vi "bats.parser.test.Multiple.SequencedUnitHeader.vi"() -> (3 "Passed":bool)   [LabVIEW 2022 SP3]
uses:
  pitch/AddOrder/AddOrderLong.Parameters.ctl
  pitch/ModifyOrder/ModifyOrderLong.Parameters.ctl
  <vilib>/Utility/error.llb/Trim Whitespace One-Sided.vi
  pitch/SequencedUnitHeader/SequencedUnitHeader.lvclass
  pitch/MessageBase/MessageBase.lvclass
  pitch/AddOrder/AddOrderLong.lvclass
  pitch/ModifyOrder/ModifyOrderLong.lvclass
panel:
  in  "ModifyOrderLong.Parameters 2":T1={"Time Offset"=0, "Order Id"="OD03", "Quantity"=0, "Price"=0.0, "Modify Flags"=0}
  in  "AddOrderLong.Parameters 2":T2={"Time Offset"=0, "Order Id"="OD02", "Quantity"=0, "Symbol"="", "Side Indicator"="", "Price"=0.0}
  in  "ModifyOrderLong.Parameters":T1={"Time Offset"=0, "Order Id"="OD02", "Quantity"=0, "Price"=0.0, "Modify Flags"=0}
  in  "AddOrderLong.Parameters":T2={"Time Offset"=0, "Order Id"="OD01", "Quantity"=0, "Symbol"="", "Side Indicator"="", "Price"=0.0}
  out "Bytes.Out.Size":i32
  out "# of Messages\nMatched?":bool[](array[boolean])
  out "Messages Matched?":bool[](array[boolean])
  out "# of SeqHdUni Matched?":bool
  in  "Expected Results":cluster{string[]}[](array[cluster])=[{["OD01", "OD02", "OD02"]}, {["OD03"]}]
  out "Results":cluster{string[]}[](array[cluster])
  out "Bytes.Out":u8[](array[numeric]) format="%.0x"
  out "Bytes.out (Visual)":u8[][](array[numeric]) format="%.0x"
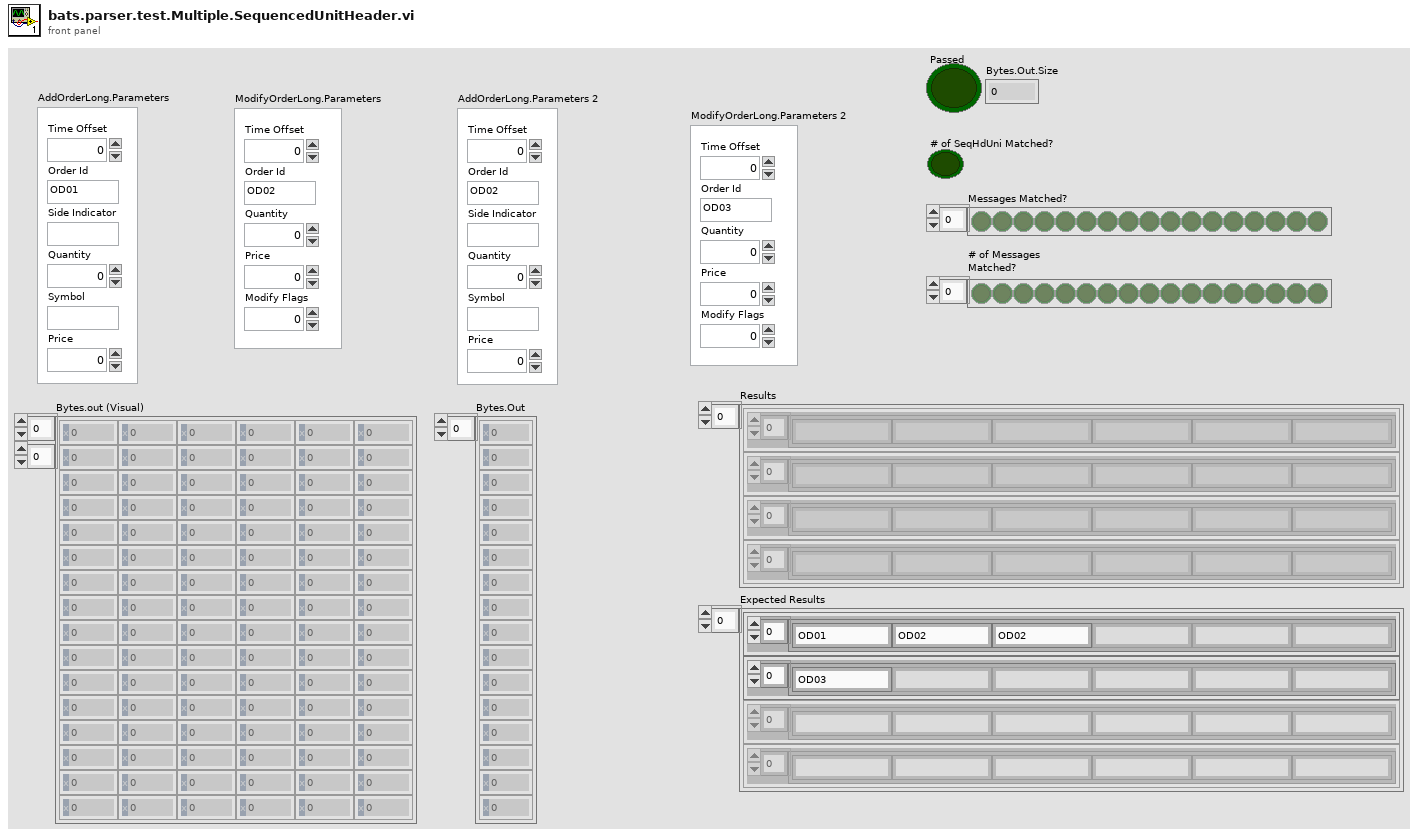
[diagram p1: front panel]
types:
  T1 = typedef "ModifyOrderLong.lvclass/ModifyOrderLong.Parameters.ctl" = cluster{"Time Offset":u32, "Order Id":string, "Quantity":u32, "Price":dbl, "Modify Flags":u8}
  T2 = typedef "AddOrderLong.lvclass/AddOrderLong.Parameters.ctl" = cluster{"Time Offset":u32, "Order Id":string, "Quantity":u32, "Symbol":string, "Side Indicator":string, "Price":dbl}
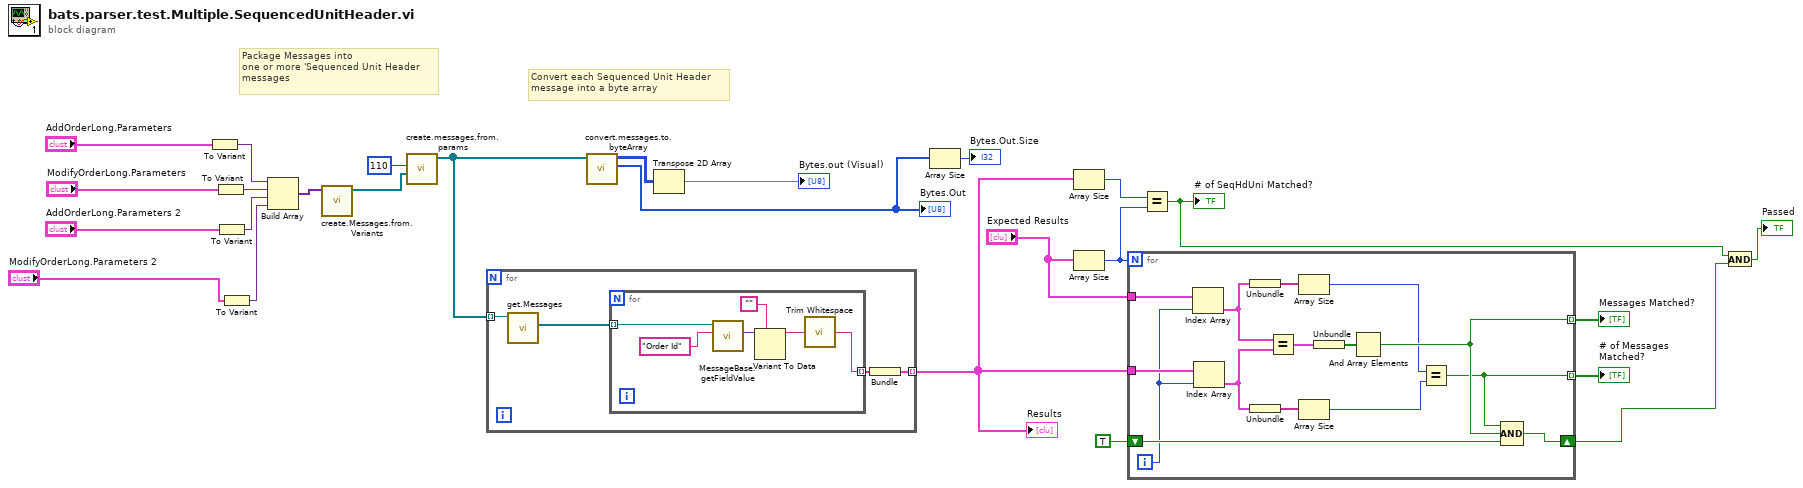
[diagram p0: block diagram]
diagram:
  # "Convert each Sequenced Unit Header\nmessage into a byte array"
  # "Package Messages into\none or more 'Sequenced Unit Header\nmessages"
  n1 = To Variant(anything="AddOrderLong.Parameters") -> (Variant=w6:variant)
  n2 = To Variant(anything="ModifyOrderLong.Parameters") -> (Variant=w5:variant)
  n3 = To Variant(anything="AddOrderLong.Parameters 2") -> (Variant=w7:variant)
  n4 = To Variant(anything="ModifyOrderLong.Parameters 2") -> (Variant=w2:variant)
  n5 = Build Array(w6, w5, w7, w2) -> (w4:variant[])
  n6 = call "create.Messages.from.Variants.vi"("Messages.Variant"=w4) -> ("Messages"=w3:refnum<class "MessageBase.lvclass">[])  [unwired: 10 in]
  n7 = call "create.messages.from.params.vi"("Message.to.Create"=w3, "Max.Frame.Size"=u16 110) -> ("Messages.Out"=w24:refnum<class "SequencedUnitHeader.lvclass">[])  [unwired: 9 in]
  n8 = for {
    tunnel: w24 -> [w30] mode=indexing
    tunnel: [w27] -> w21 mode=indexing
    n9 = call-dynamic "get.Messages.vi"("SequencedUnitHeader in"=w30) -> ("Messages.Out"=w29:refnum<class "MessageBase.lvclass">[])  [unwired: 8 in, 2 out]
    n10 = for {
      tunnel: w29 -> [w34] mode=indexing
      tunnel: [w31] -> w28 mode=indexing
      n11 = call-dynamic "MessageBase.getFieldValue.vi"("FIeld.Name"="Order Id" ("Field.Name"), "MessageBase in"=w34) -> ("FieldValue"=w33:variant)  [unwired: 7 in, 2 out]
      n12 = Variant To Data(type="", Variant=w33) -> (data=w32:string)  [unwired: 1 in, 1 out]
      n13 = call <vilib>:"Trim Whitespace.vi"("string"=w32) -> ("trimmed string"=w31:string)  [unwired: 1 in]
    }
    n14 = Bundle(w28) -> (w27:cluster{string[]})  [unwired: 1 in]
  }
  "Results" <- w21
  n15 = call "convert.messages.to.byteArray.vi"("Messages.In"=w24) -> ("ByteArray.out"=w13:u8[], "2D.ByteArray.out"=w26:u8[][])  [unwired: 9 in]
  "Bytes.Out" <- w13
  n16 = Transpose 2D Array(2D array=w26) -> (transposed array=→"Bytes.out (Visual)":u8[][])
  n17 = Array Size(array=w13) -> (size(s)=→"Bytes.Out.Size":i32)
  n18 = Array Size(array=w21) -> (size(s)=w19:i32)
  n19 = Array Size(array="Expected Results") -> (size(s)=w20:i32)
  n20 = for {
    N: w20 -> [_]
    shift-right: [w50] -> w16
    shift-left: TRUE -> [w51]
    tunnel: w21 -> [w49]
    tunnel: "Expected Results" -> [w48]
    tunnel: [w44] -> w18 mode=indexing
    tunnel: [w37] -> w17 mode=indexing
    i -> [w47]
    n21 = Index Array(array=w48, index=w47) -> (element=w43:cluster{string[]})
    n22 = Index Array(array=w49, index=w47) -> (element=w42:cluster{string[]})
    n23 = Unbundle(w43) -> (w40:string[])
    n24 = Unbundle(w42) -> (w41:string[])
    n25 = Equal?(x=w43, y=w42) -> (x = y?=w46:cluster{bool[]})
    n26 = Array Size(array=w40) -> (size(s)=w39:i32)
    n27 = Array Size(array=w41) -> (size(s)=w38:i32)
    n28 = Unbundle(w46) -> (w45:bool[])
    n29 = And Array Elements(Boolean array=w45) -> (logical AND=w44:bool)
    n30 = Equal?(x=w39, y=w38) -> (x = y?=w37:bool)
    n31 = Compound Arithmetic op=AND(w37, w44, w51) -> (w50:bool)
  }
  "Messages Matched?" <- w18
  "# of Messages\nMatched?" <- w17
  n32 = Equal?(x=w19, y=w20) -> (x = y?=w15:bool)
  "# of SeqHdUni Matched?" <- w15
  n33 = And(x=w15, y=w16) -> (x .and. y?=→"Passed":bool)
